vi "Parse Results (all).vi"(6 "Type":T1, 8 "error in (no error)":errorcluster, 11 "Results (Dictionary)":cluster{"key":string, "value":dbl}[](array[cluster])) -> (0 "error out":errorcluster, 1 "Names":string[](array[string]), 2 "Data":dbl[](array[numeric]), 3 "Results (Dictionary)":cluster{"key":string, "value":dbl}[](array[cluster]))   [LabVIEW 2019, in "Instrument.Lockin.lvclass"]
uses:
  Instrument.Lockin.lvclass
  Typedefs/Results Type--Enum.ctl
  <userlib>/_OpenG.lib/array/array.llb/Remove Duplicates from 1D Array (I32)__ogtk.vi
  <userlib>/_OpenG.lib/array/array.llb/Delete Elements from 1D Array (String)__ogtk.vi
  <userlib>/_OpenG.lib/array/array.llb/Index 1D Array Elements (DBL)__ogtk.vi
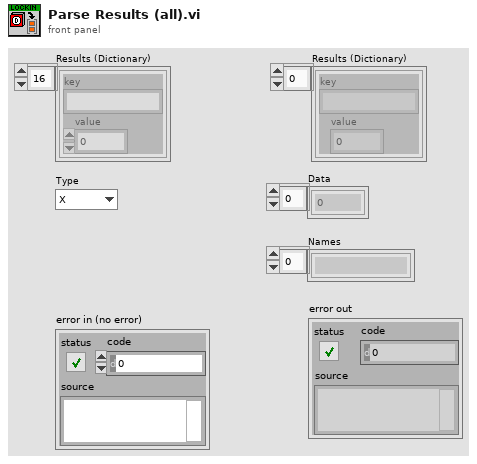
[diagram p1: front panel]
types:
  T1 = typedef "Instrument.Lockin.lvclass/Results Type--Enum.ctl" = enum16{"X", "Y", "R", "Theta", "Mean"}
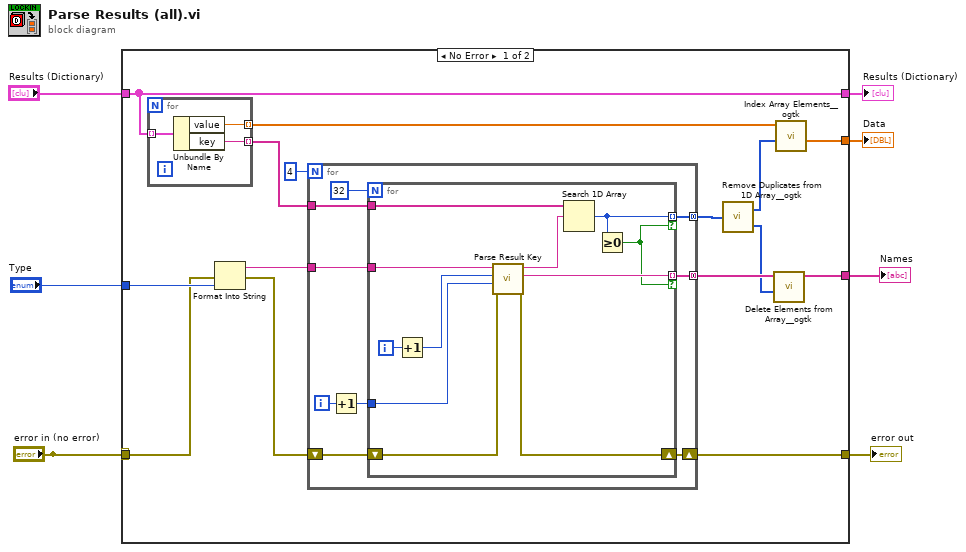
[diagram p0: block diagram]
diagram:
  n1 = case shown="No Error" "error in (no error)" {
    selector: "error in (no error)" -> [_ w46]
    tunnel: [w19 _] -> w7
    tunnel: "Type" -> [w16 _]
    tunnel: "Results (Dictionary)" -> [w17 w47]
    tunnel: [w8 _] -> w4
    tunnel: [w18 w46] -> w3
    tunnel: [w17 w47] -> w2
    tunnel: "error in (no error)" -> [w14 _]
    frame No Error {
      n2 = for {
        tunnel: [w45] -> w22 mode=indexing
        tunnel: [w44] -> w21 mode=indexing
        tunnel: w17 -> [w43] mode=indexing
        n3 = Unbundle By Name(w43) -> ("value"=w45:dbl, "key"=w44:string)
      }
      n4 = Format Into String(error in=w14, w16) -> (resulting string=w15:string, error out=w13:errorcluster)  [unwired: 2 in]
      n5 = for {
        N: 4 ("Numeric") -> [_]
        tunnel: w15 -> [w31]
        tunnel: [w30] -> w12 mode=concatenating
        tunnel: w21 -> [w29]
        tunnel: [w26] -> w11 mode=concatenating
        shift-right: [w23] -> w18
        shift-left: w13 -> [w24]
        i -> [w25]
        n6 = Increment(x=w25) -> (x+1=w27:i32)
        n7 = for {
          N: 32 -> [_]
          tunnel: w29 -> [w40]
          tunnel: w31 -> [w42]
          tunnel: [w38] -> w30 mode=indexing if=w32
          tunnel: w27 -> [w33]
          tunnel: [w37] -> w26 mode=indexing if=w32
          shift-right: [w35] -> w23
          shift-left: w24 -> [w36]
          i -> [w41]
          n8 = Increment(x=w41) -> (x+1=w34:i32)
          n9 = call "Parse Result Key.vi"("error in (no error)"=w36, "Ref Channel"=w33, "AI Channel"=w34, "Datatype"=w42) -> ("error out"=w35:errorcluster, "Label"=w37:string, "Key"=w39:string)  [unwired: 5 in]
          n10 = Search 1D Array(1D array=w40, element=w39) -> (index of element=w38:i32)  [unwired: 1 in]
          n11 = Greater Or Equal To 0?(x=w38) -> (x >= 0?=w32:bool)
        }
      }
      n12 = call-poly <userlib>:"Remove Duplicates from 1D Array__ogtk.vi"("Input Array"=w12) -> ("Output Array"=w10:i32[], "indices of removed elements"=w9:i32[])
      n13 = call-poly <userlib>:"Delete Elements from Array__ogtk.vi"("indices"=w9, "array"=w11) -> ("array w/ subset deleted"=w8:string[])  [unwired: 8 in, 1 out]
      n14 = call-poly <userlib>:"Index Array Elements__ogtk.vi"("indices"=w10, "array"=w22) -> ("elements"=w19:dbl[])  [unwired: 9 in]
    }
    frame Error {
    }
  }
  "Data" <- w7
  "Results (Dictionary)" <- w2
  "Names" <- w4
  "error out" <- w3
